vi "Read Default Test Strategies.vi"(11 "Banana in":refnum<class "Banana.lvclass">) -> (1 "Strategies":T1, 3 "Banana out":refnum<class "Banana.lvclass">)   [LabVIEW 2021, in "Bananas.lvlib" / "Banana.lvclass"]
uses:
  Banana.lvclass
  Test Strategies -- cluster.ctl
  DefineTest/DefineTest.lvclass
  Banana.lvclass/Banana.ctl
  <vilib>/LabVIEW Open Source Project/Data Manipulation/Variant/Variant_EmptyCluster.vi
  <vilib>/LabVIEW Open Source Project/Data Manipulation/TypeDescriptor/TypeDescriptor_SetName.vi
  <vilib>/Utility/GetType.llb/TD_Create Cluster.vi
  <vilib>/LabVIEW Open Source Project/Data Manipulation/Variant/OpenVariant.lvlib
  Bananas.lvlib
  BananaPeel/BananaPeel.lvclass
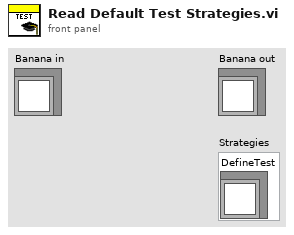
[diagram p1: front panel]
types:
  T1 = typedef "Bananas.lvlib/Test Strategies -- cluster.ctl" = cluster{"DefineTest":refnum<class "DefineTest.lvclass">}
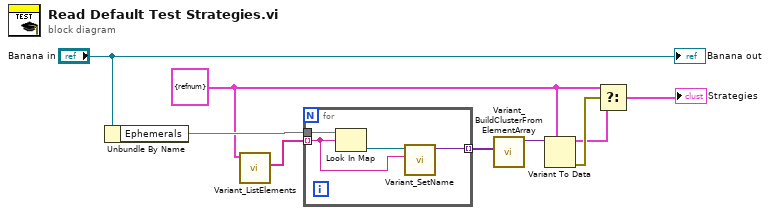
[diagram p0: block diagram]
diagram:
  w1 = T1 {"DefineTest"=refnum} ("Strategies")
  n1 = Unbundle By Name("Banana in") -> ("Ephemerals"=w7:map{string, refnum<class "BananaPeel.lvclass">})
  n2 = call <vilib>:"Variant_ListElements.vi"("Variant"=w1) -> ("element names"=w8:string[])  [unwired: 7 in, 3 out]
  n3 = for {
    tunnel: w7 -> [w13]
    tunnel: w8 -> [w10] mode=indexing
    tunnel: [w11] -> w6 mode=indexing
    n4 = Look In Map(map=w13, key=w10) -> (value=w12:refnum<class "BananaPeel.lvclass">)  [unwired: 1 in, 1 out]
    n5 = call <vilib>:"Variant_SetName.vi"("Name"=w10, "Variant"=w12) -> ("Named Variant"=w11:variant)  [unwired: 9 in]
  }
  n6 = call <vilib>:"Variant_BuildClusterFromElementArray.vi"("Elements"=w6) -> ("Cluster"=w5:variant)  [unwired: 10 in]
  n7 = Variant To Data(type=w1, Variant=w5) -> (data=w3:T1, error out=w4:errorcluster)  [unwired: 1 in]
  n8 = Select(t=w1, s=w4, f=w3) -> (s? t:f=→"Strategies":T1)
  "Banana out" <- "Banana in"
